vi "USRP Packet Transmitter_Global.vi"() -> ()   [LabVIEW 2013]
uses:
  <vilib>/addons/Modulation/Digital/General/MT Generate PSK System Parameters(M).vi
  Global 1.vi
  <vilib>/addons/Modulation/niDMT.lvlib
panel:
  in  "stop":bool
  out "Constellation Graph":T1(graph)
  out "Transmitted Signal":cluster{"t0":dbl, "dt":dbl, "Y":dbl[]}(graph)
  in  "Sample Rate [s/sec]":dbl=400000.0 format="%#.6p"
  in  "Modulation type":string(combo)="QPSK"
  in  "Pulse Shaping\nFilter Parameters":T2={"Alpha"=0.5, "Filter Length"=6, "TX Filter"=enum."Root Raised Cos"} caption="Pulse Shaping Filter" {"Alpha" format="%.2f"}
  out "Symbol Rate [symbols/sec]":dbl=50000.0 format="%#.6p"
  in  "Message Text":string="Two roads diverged in a yellow wood,\nAnd sorry I could not travel both\nAnd be one traveler, long I stood\nAnd looked down one as far as I could\nTo where it bent in the undergrowth.\n\nThen took the other, as just as fair,\nAnd having perhaps the better claim,\nBecause it was grassy and wanted wear;\nThough as for that the passing there\nHad worn them really about the same.\n\nAnd both that morning equally lay\nIn leaves no step had trodden black.\nOh, I kept the first for another day!\nYet knowing how way leads on to way,\nI doubted if I should ever come back.\n\nI shall be telling this with a sigh\nSomewhere ages and ages hence:\nTwo roads diverged in a wood, and I--\nI took the one less traveled by,\nAnd that has made all the difference.\n"
  in  "Packet Parameters":T3={"Guard Bits "=30, "Sync Bits"=20, "Message Bits"=128}
  in  "Packet Pad [samples]":i32=200
  in  "16-PSK System Parameters":T4={"Samples per Symbol"=8, "symbol map"=[], "Differential PSK"=enum."disable", "PSK type"=0} {"PSK type" items=["normal", "shifted", "offset"]; "symbol map" format="%.3f"}
  in  "8-PSK System Parameters":T4={"Samples per Symbol"=8, "symbol map"=[], "Differential PSK"=enum."disable", "PSK type"=0} {"PSK type" items=["normal", "shifted", "offset"]; "symbol map" format="%.3f"}
  in  "QPSK System Parameters":T4={"Samples per Symbol"=8, "symbol map"=[], "Differential PSK"=enum."disable", "PSK type"=0} {"PSK type" items=["normal", "shifted", "offset"]; "symbol map" format="%.3f"}
  in  "BPSK System Parameters":T4={"Samples per Symbol"=8, "symbol map"=[], "Differential PSK"=enum."disable", "PSK type"=0} {"PSK type" items=["normal", "shifted", "offset"]; "symbol map" format="%.3f"}
  out "Number of Packets in Message":i32=46
  in  "PN sequence order\n for Sync Bits":i32=31 caption="PN sequence order (9)"
  in  "Message Type":bool=TRUE
  # "Pad\nData"
  # "Guard\nBand"
  # "Sync\nSeq"
  # "Packet\nNumber"
  # "Data"
  # "Custom Text"
  # "PN Sequence"
  # "Cyclic Pad"
  # "Guard\nBand"
  # "Sync\nSeq"
  # "Packet\nNumber"
  # "Data"
  # "Packet Transmitter"
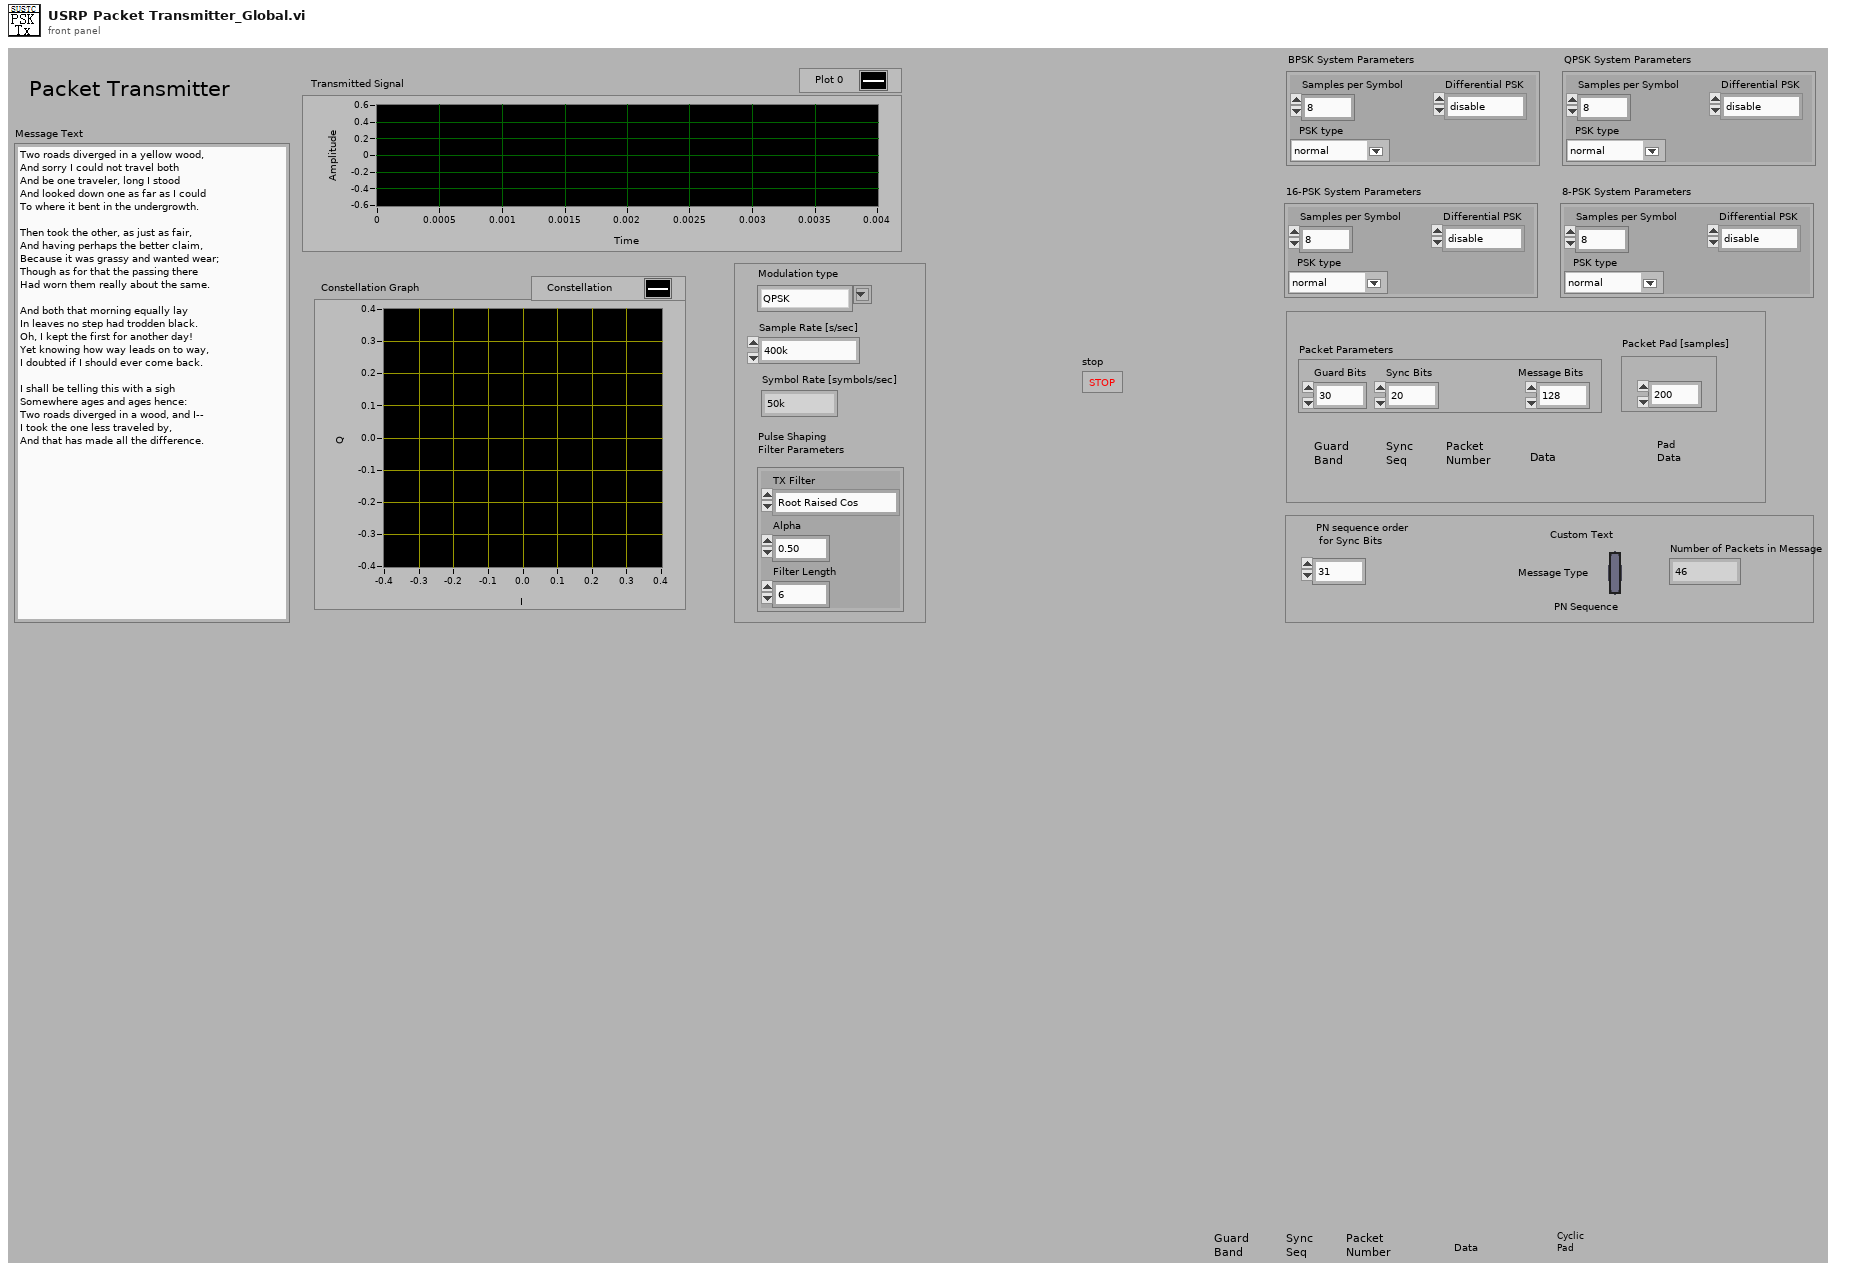
[diagram p1: front panel]
types:
  T1 = cluster{"constellation":dbl[], "oversampled data":dbl[]}[]
  T2 = cluster{"Alpha":dbl, "Filter Length":i32, "TX Filter":enum16{"none", "Raised Cosine", "Root Raised Cos", "Gaussian"}}
  T3 = cluster{"Guard Bits ":i32, "Sync Bits":i32, "Message Bits":i32}
  T4 = cluster{"Samples per Symbol":i32, "symbol map":cdb[], "Differential PSK":enum16{"disable", "enable"}, "PSK type":u16}
  T5 = cluster{"samples per symbol (16)":i32, "symbol map":cdb[], "differential PSK":enum16{"disable", "enable"}, "PSK type":u16}
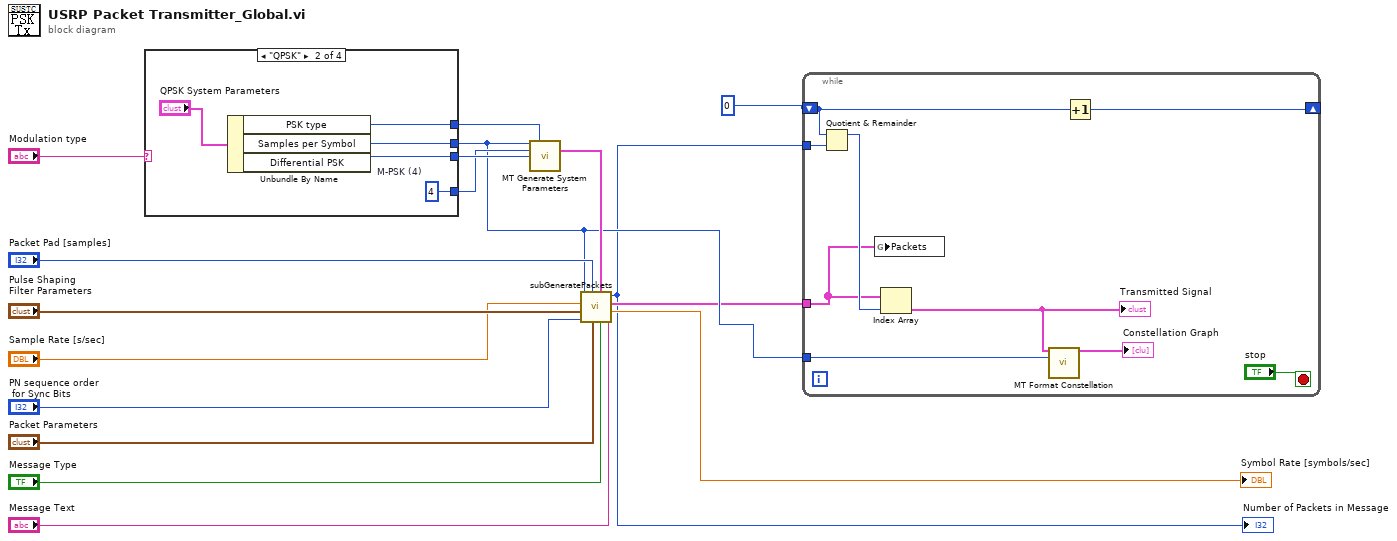
[diagram p0: block diagram]
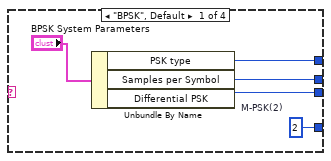
[diagram p2: hidden frame]
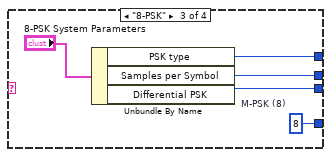
[diagram p3: hidden frame]
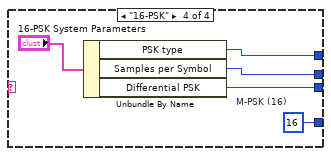
[diagram p4: hidden frame]
diagram:
  n1 = case shown="\"QPSK\"" "Modulation type" {
    tunnel: [w19 w23 w31 w37] -> w3
    tunnel: [w20 w25 w30 w36] -> w17
    tunnel: [w22 w27 w29 w35] -> w15
    tunnel: [w21 w26 w32 w34] -> w11
    frame "BPSK", Default {
      w22 = 2  # M-PSK(2)
      n2 = Unbundle By Name("BPSK System Parameters") -> ("PSK type"=w21:u16, "Samples per Symbol"=w19:i32, "Differential PSK"=w20:enum16{"disable", "enable"})
    }
    frame "QPSK" {
      w27 = 4  # M-PSK (4)
      n3 = Unbundle By Name("QPSK System Parameters") -> ("PSK type"=w26:u16, "Samples per Symbol"=w23:i32, "Differential PSK"=w25:enum16{"disable", "enable"})
    }
    frame "8-PSK" {
      w29 = 8  # M-PSK (8)
      n4 = Unbundle By Name("8-PSK System Parameters") -> ("PSK type"=w32:u16, "Samples per Symbol"=w31:i32, "Differential PSK"=w30:enum16{"disable", "enable"})
    }
    frame "16-PSK" {
      w35 = 16  # M-PSK (16)
      n5 = Unbundle By Name("16-PSK System Parameters") -> ("PSK type"=w34:u16, "Samples per Symbol"=w37:i32, "Differential PSK"=w36:enum16{"disable", "enable"})
    }
  }
  n6 = call-poly <vilib>:"MT Generate System Parameters.vi"("samples per symbol (16)"=w3, "PSK type"=w11, "M-PSK (4)"=w15, "differential PSK"=w17) -> ("PSK system parameters"=w12:T5)  [unwired: 9 in, 2 out]
  n7 = call "subGeneratePackets.vi"("Message Text"="Message Text", "Message Type"="Message Type", "PSK system parameters"=w12, "Packet Parameters"="Packet Parameters", "Packet Pad \n[samples]"="Packet Pad [samples]", "PN sequence order\nfor Sync Bits"="PN sequence order\n for Sync Bits", "Pulse Shaping Filter Parameters"="Pulse Shaping\nFilter Parameters", "Tx IQ Sampling\nRate [s/sec]"="Sample Rate [s/sec]", "Samples per Symbol"=w3) -> ("Symbol Rate"=→"Symbol Rate [symbols/sec]":dbl, "Packets"=w2:cluster{"t0":dbl, "dt":dbl, "Y":cdb[]}[], "Number of Packets"=w1:i32)
  "Number of Packets in Message" <- w1
  n8 = while {
    shift-right: [w43] -> _
    shift-left: 0 -> [w39]
    tunnel: w3 -> [w42]
    tunnel: w2 -> [w41]
    tunnel: w1 -> [w40]
    stop <- "stop" stop-if-true
    n9 = Quotient & Remainder(x=w39, y=w40) -> (x-y*floor(x/y)=w46:i32)  [unwired: 1 out]
    n10 = global write "Global 1.vi" "Packets"(w41) -> ()
    n11 = Index Array(array=w41, index=w46) -> (element=w45:cluster{"t0":dbl, "dt":dbl, "Y":cdb[]})
    "Transmitted Signal" <- w45
    n12 = call <vilib>:"MT Format Constellation.vi"("waveform"=w45, "samples per symbol"=w42) -> ("constellation graph"=→"Constellation Graph":T1)  [unwired: 12 in, 1 out]
    n13 = Increment(x=w39) -> (x+1=w43:i32)
  }
